vi "FM_RTL-SDR_RX_atan2_NET_X64.vi"() -> (3 "Calculation Time (s)":dbl)   [LabVIEW 2013]
doc: "Demonstrates how to use the MATLAB script node. The m-file script is used to calculate the data and the resulting fractal is displayed on the front panel. The MathWorks, Inc. MATLAB (R) Application Software version 5.0 or later must be installed and properly licensed in order to run this VI."
uses:
  6.3_DLL_X64/FMDemod/NET/FMDemodRTLSDR_NET/for_testing/FMDemodRTLSDR_NET.dll
  <vilib>/Waveform/WDTFileIO.llb/Read Waveform from File.vi
panel:
  out "size(s)":i32
  out "Baseband":dbl[](array[numeric])
  in  "file path":path=path "D:/File/Recoder_Data_IQIQ"
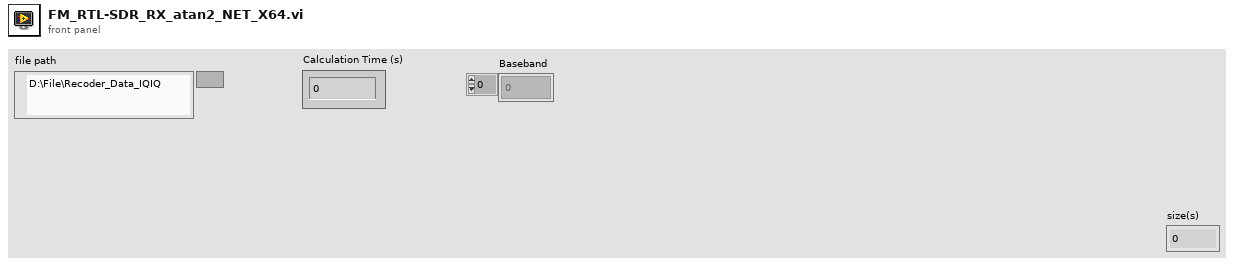
[diagram p1: front panel]
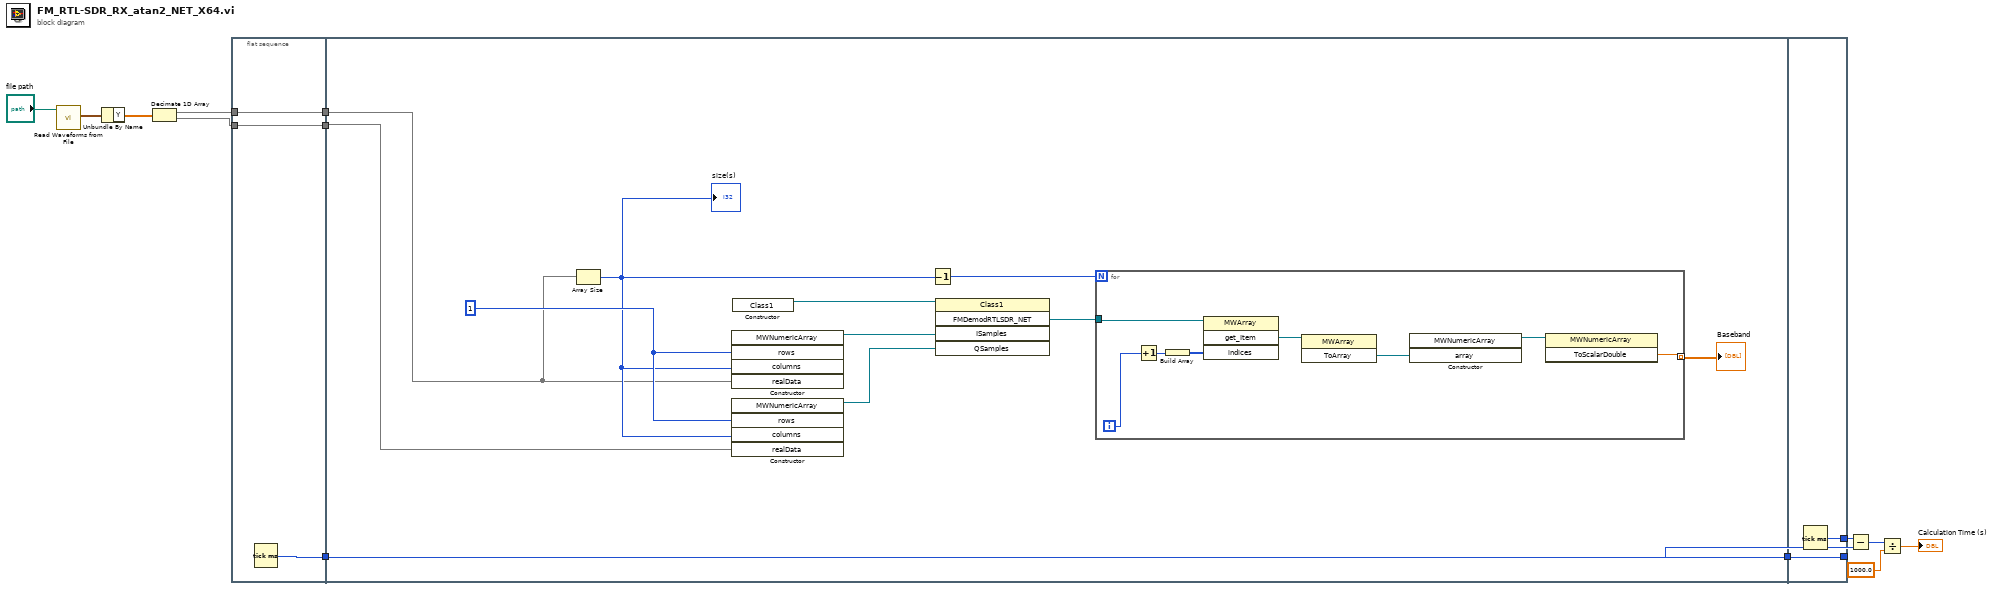
[diagram p0: block diagram]
diagram:
  n1 = call-poly <vilib>:"Read Waveforms from File.vi"("file path (dialog if empty)"="file path") -> ("first waveform in record"=w7:waveform(dbl))  [unwired: 5 in, 3 out]
  n2 = Unbundle By Name(w7) -> ("Y"=w5:dbl[])
  n3 = Decimate 1D Array(w5) -> (w2:dbl[], w1:dbl[])
  n4 = flat-sequence {
    tunnel: [w17] -> w8
    tunnel: [w16] -> w4
    tunnel: w2 -> [w16]
    tunnel: [w15] -> w3
    tunnel: w1 -> [w15]
    tunnel: [w28] -> w14
    tunnel: w8 -> [w28]
    tunnel: w4 -> [w21]
    tunnel: w3 -> [w20]
    tunnel: w14 -> [w37]
    tunnel: [w38] -> w11
    tunnel: [w37] -> w10
    frame #0 {
      n5 = Tick Count (ms)() -> (millisecond timer value=w17:u32)
    }
    frame #1 {
      w24 = 1 ("rows")
      n6 = Array Size(array=w21) -> (size(s)=w22:i32)
      "size(s)" <- w22
      n7 = constructor class="MWNumericArray"("rows"=w24, "columns"=w22, "realData"=w21) -> (reference out=w26:refnum<k24>)  [unwired: 3 in, 5 out]
      n8 = constructor class="MWNumericArray"("rows"=w24, "columns"=w22, "realData"=w20) -> (reference out=w25:refnum<k24>)  [unwired: 3 in, 5 out]
      n9 = constructor class="Class1"() -> (reference out=w27:refnum<k24>)  [unwired: 3 in, 2 out]
      n10 = Decrement(x=w22) -> (x-1=w23:i32)
      n11 = invoke class="Class1" method="FMDemodRTLSDR_NET"(reference=w27, "ISamples"=w26, "QSamples"=w25) -> ("FMDemodRTLSDR_NET"=w18:refnum<k24>)  [unwired: 2 in, 4 out]
      n12 = for {
        N: w23 -> [_]
        tunnel: [w30] -> w19 mode=indexing
        tunnel: w18 -> [w29]
        i -> [w36]
        n13 = Increment(x=w36) -> (x+1=w35:i32)
        n14 = Build Array(w35) -> (w34:i32[])
        n15 = invoke class="MWArray" method="get_Item"(reference=w29, "indices"=w34) -> ("get_Item"=w33:refnum<k24>)  [unwired: 2 in, 3 out]
        n16 = invoke class="MWArray" method="ToArray"(reference=w33) -> ("ToArray"=w32:refnum<k24>)  [unwired: 2 in, 2 out]
        n17 = constructor class="MWNumericArray"("array"=w32) -> (reference out=w31:refnum<k24>)  [unwired: 3 in, 3 out]
        n18 = invoke class="MWNumericArray" method="ToScalarDouble"(reference=w31) -> ("ToScalarDouble"=w30:dbl)  [unwired: 2 in, 2 out]
      }
      "Baseband" <- w19
    }
    frame #2 {
      n19 = Tick Count (ms)() -> (millisecond timer value=w38:u32)
    }
  }
  n20 = Subtract(x=w11, y=w10) -> (x-y=w12:u32)
  n21 = Divide(x=w12, y=1000.0) -> (x/y=→"Calculation Time (s)":dbl)
